vi "Load JSON Templates.vi"() -> (2 "JSON Template Names":string[](array[string]), 3 "JSON Templates":refnum<class "JSON Routing Channel Template.lvclass">[](array[class]))   [LabVIEW 2020, in "Routing and Faulting System Explorer.lvlib"]
uses:
  Routing and Faulting System Explorer.lvlib
  Routing Templates/Routing Channel Templates/JSON Routing Channel Template/JSON Routing Channel Template.lvclass
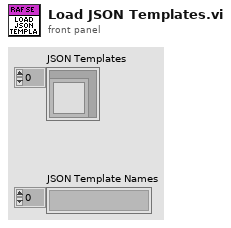
[diagram p1: front panel]
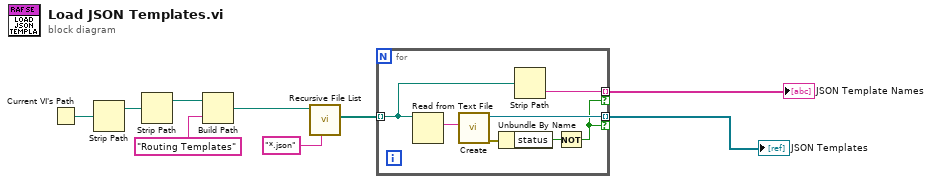
[diagram p0: block diagram]
diagram:
  n1 = Current VI's Path() -> (path=w1:path)
  n2 = Strip Path(path=w1) -> (stripped path=w2:path)  [unwired: 1 out]
  n3 = Strip Path(path=w2) -> (stripped path=w3:path)  [unwired: 1 out]
  n4 = Build Path(base path=w3, name or relative path="Routing Templates") -> (appended path=w5:path)
  n5 = call <vilib>:"Recursive File List.vi"("pattern"="*.json", "Folder Path"=w5) -> ("All Files in Dir"=w7:path[])  [unwired: 5 in, 4 out]
  n6 = for {
    tunnel: w7 -> [w11] mode=indexing
    tunnel: [w15] -> w9 mode=indexing if=w12
    tunnel: [w10] -> w8 mode=indexing if=w12
    n7 = Read from Text File(file (use dialog)=w11) -> (text=w16:string)  [unwired: 3 in, 3 out]
    n8 = call "Create.vi"("JSON"=w16) -> ("error out"=w14:errorcluster, "JSON Routing Channel Template out"=w15:refnum<class "JSON Routing Channel Template.lvclass">)  [unwired: 9 in]
    n9 = Unbundle By Name(w14) -> ("status"=w13:bool)
    n10 = Strip Path(path=w11) -> (name=w10:string)  [unwired: 1 out]
    n11 = Not(x=w13) -> (.not. x?=w12:bool)
  }
  "JSON Templates" <- w9
  "JSON Template Names" <- w8
